vi "参考灵敏度测试.vi"(6 "参数":string, 7 "模板":refnum<class "NI_report.lvclass">, 8 "参考通道":tag, 9 "被测通道":tag, 10 "33XXX":refnum<visa-resource-name>) -> (0 "错误输出":errorcluster)   [LabVIEW 2015]
uses:
  <vilib>/Utility/NIReport.llb/NI_report.lvclass
  Global.vi
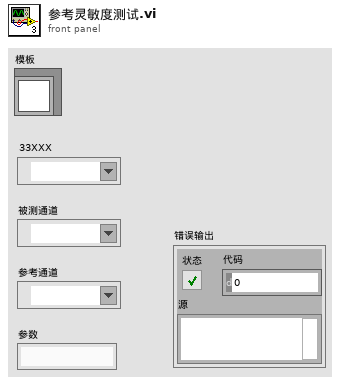
[diagram p1: front panel]
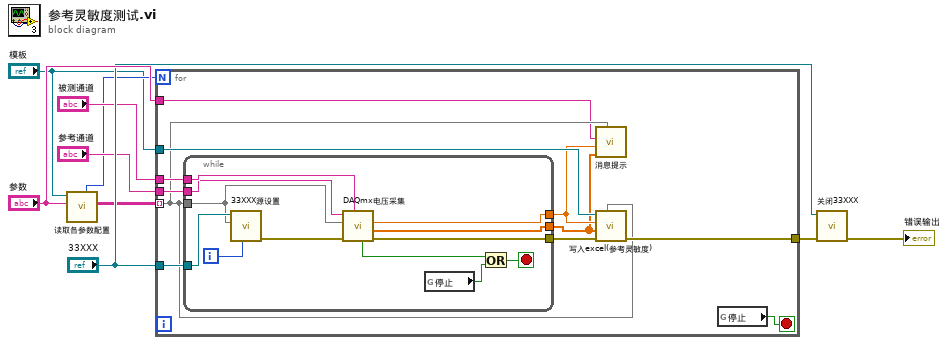
[diagram p0: block diagram]
diagram:
  n1 = call "读取各参数配置.vi"("参数"="参数", "NI_report输入"="模板") -> ("设置"=w3:string[][], "测量点数"=w2:i32)  [unwired: 6 in, 2 out]
  n2 = for {
    N: w2 -> [_]
    tunnel: w3 -> [w14] mode=indexing
    tunnel: "33XXX" -> [w20]
    tunnel: "被测通道" -> [w19]
    tunnel: "参考通道" -> [w18]
    tunnel: "模板" -> [w17]
    tunnel: [w15] -> w6
    tunnel: "参数" -> [w13]
    stop <- w11 stop-if-true
    n3 = while {
      tunnel: w14 -> [w27]
      tunnel: w20 -> [w31]
      tunnel: w19 -> [w30]
      tunnel: w18 -> [w29]
      tunnel: [w26] -> w12
      tunnel: [w25] -> w10
      tunnel: [w24] -> w16
      i -> [w32]
      stop <- w21 stop-if-true
      n4 = call "33XXX源设置.vi"("步长"=w32, "设置"=w27, "VISA引用句柄输入"=w31) -> ("error out"=w28:errorcluster)  [unwired: 7 in, 1 out]
      n5 = call "DAQmx电压采集.vi"("被测通道"=w30, "error in"=w28, "设置"=w27, "参考通道"=w29) -> ("error out"=w24:errorcluster, "被测幅值"=w25:dbl[], "参考幅值"=w26:dbl, "满足条件"=w23:bool)  [unwired: 4 in]
      n6 = global read "Global.vi" "停止"() -> (w22:bool)
      n7 = Or(x=w23, y=w22) -> (x .or. y?=w21:bool)
    }
    n8 = call "消息提示.vi"("设置"=w14, "被测幅值"=w10, "参考幅值"=w12, "参数"=w13) -> ()  [unwired: 8 in]
    n9 = call "写入excel(参考灵敏度).vi"("设置"=w14, "error in (no error)"=w16, "被测幅值"=w10, "参考幅值"=w12, "NI_report输入"=w17) -> ("error out"=w15:errorcluster)  [unwired: 5 in, 1 out]
    n10 = global read "Global.vi" "停止"() -> (w11:bool)
  }
  n11 = call "关闭33XXX.vi"("error in"=w6, "VISA引用句柄输入"="33XXX") -> ("error out"=→"错误输出":errorcluster)  [unwired: 8 in, 1 out]
